vi "synchronize device.vi"(8 "error in (no error)":errorcluster, 11 "Template in":refnum<class "Template.lvclass">) -> (0 "error out":errorcluster, 3 "Template out":refnum<class "Template.lvclass">)   [LabVIEW 2020, in "Template.lvlib" / "Template.lvclass"]
uses:
  Template.lvclass
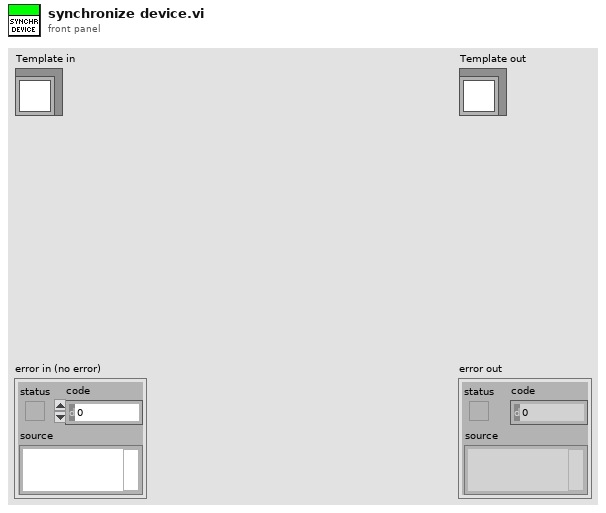
[diagram p1: front panel]
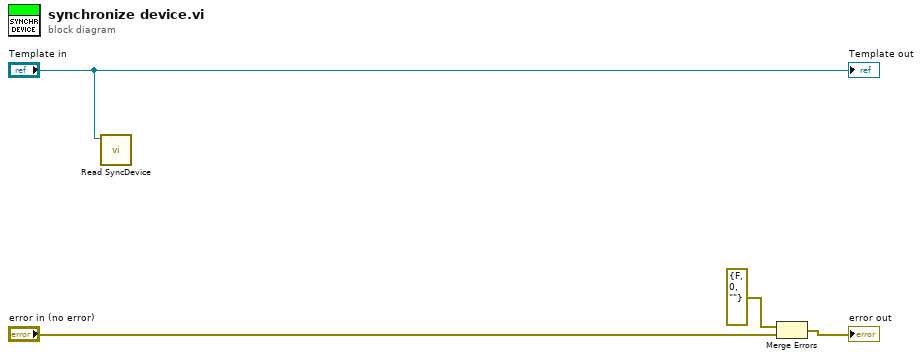
[diagram p0: block diagram]
diagram:
  n1 = call "Read SyncDevice.vi"("Template in"="Template in") -> ()  [unwired: 10 in, 1 out]
  n2 = Merge Errors(errorcluster {"status"=FALSE, "code"=0, "source"=""} ("error in"), "error in (no error)") -> (→"error out":errorcluster)
  "Template out" <- "Template in"
